vi "m1m3_monitorCommand_EnableHardpointChase.vi"(8 "error in (no error)":errorcluster, 11 "command_EnableHardpointChase_Ctl":T1) -> (0 "error out":errorcluster, 2 "function return":i32, 3 "command_EnableHardpointChase_Ctl out":T1)   [LabVIEW 2016, in "SALLV_m1m3.lvlib"]
doc: "int m1m3_shm_monitorCommand_EnableHardpointChaseLV(m1m3_command_EnableHardpointChaseLV *command_EnableHardpointChase_Ctl );"
uses:
  SALLV_m1m3.lvlib
  DataTypes/command_EnableHardpointChase.ctl
  SALLV_m1m3.so
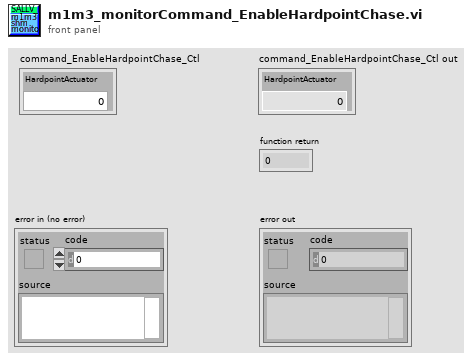
[diagram p1: front panel]
types:
  T1 = typedef "SALLV_m1m3.lvlib/command_EnableHardpointChase.ctl" = cluster{"HardpointActuator":i32}
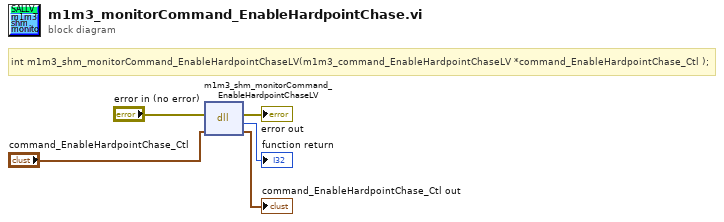
[diagram p0: block diagram]
diagram:
  # "int m1m3_shm_monitorCommand_EnableHardpointChaseLV(m1m3_command_EnableHardpointChaseLV *command_EnableHardpointChase_Ctl );"
  n1 = dll-call lib="opt/CODE/SALLV_m1m3/SALLV_m1m3.*" fn="m1m3_shm_monitorCommand_EnableHardpointChaseLV"(error in="error in (no error)", "command_EnableHardpointChase_Ctl"="command_EnableHardpointChase_Ctl") -> (error out=→"error out":errorcluster, →"function return":i32, "command_EnableHardpointChase_Ctl"=→"command_EnableHardpointChase_Ctl out":T1)  [unwired: 2 in, 1 out]
